vi "Tosca-Initialize Hardware.vi"(0 "Tosca":refnum<class "Parameters.lvclass">, 11 "error in (no error)":errorcluster) -> (4 "Tosca out":refnum<class "Parameters.lvclass">, 14 "SG Runtime":T1, 15 "error out":errorcluster)   [LabVIEW 2020]
uses:
  Typedefs/Tosca-SG Runtime Params.ctl
  Typedefs/Tosca-AO Runtime.ctl
  Typedefs/Tosca-DO Runtime.ctl
  Imaging VIs/Tosca-Imaging Mode.ctl
  Classes/Parameters/Parameters.lvclass
  epl-vi-lib/PXI DAQ VIs/AODO/Typedefs/AODO-Config.ctl
  epl-vi-lib/PXI DAQ VIs/AODO/Typedefs/AODO-Output Spec.ctl
  epl-vi-lib/PXI DAQ VIs/AODO/Typedefs/DO-Output Spec.ctl
  epl-vi-lib/PXI DAQ VIs/AODO/Typedefs/AODO-Action.ctl
  Imaging VIs/Tosca-2P Config.ctl
  Classes/Parameters/Parameters.lvclass/Parameters.ctl
  Classes/Parameters/Read Imaging.vi
  Classes/Parameters/Read DAQ.vi
  Tosca-Globals.vi
  epl-vi-lib/Utility VIs/File IO VIs/Configuration File Wrapper VIs/Config-Read Key (string).vi
  epl-vi-lib/Utility VIs/Array Manipulation VIs/Sort and Index (string).vi
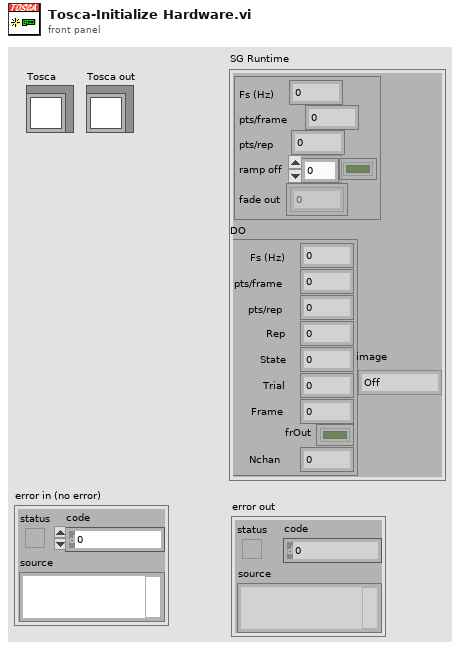
[diagram p1: front panel]
types:
  T1 = typedef "Tosca-SG Runtime Params.ctl" = cluster{"AO":T2, "DO":T3, "image":T4}
  T2 = typedef "Tosca-AO Runtime.ctl" = cluster{"Fs (Hz)":dbl, "pts/frame":i32, "pts/rep":i32, "ramp off":bool[], "fade out":dbl[][]}
  T3 = typedef "Tosca-DO Runtime.ctl" = cluster{"Fs (Hz)":dbl, "pts/frame":i32, "pts/rep":i32, "Rep":i32, "State":i32, "Trial":i32, "Frame":i32, "frOut":bool[], "Nchan":i32}
  T4 = typedef "Tosca-Imaging Mode.ctl" = enum16{"Off", "Widefield", "Two-photon"}
  T5 = typedef "AODO-Action.ctl" = enum16{"Configure", "Initialize", "Start", "Write", "Clean up", "Init & Start", "Config & Test", "Position", "Set AO Gains", "Zero", "Prime", "Status"}
  T6 = typedef "AODO-Config.ctl" = cluster{"AO":T7, "DO":T8, "hold outputs":bool, "ExtTrig":bool, "Trig Src":string, "regen":bool, "finite":bool}
  T7 = typedef "AODO-Output Spec.ctl" = cluster{"Channels":string[], "Fs (Hz)":dbl, "Npts":i32, "Gains":dbl[]}
  T8 = typedef "DO-Output Spec.ctl" = cluster{"Channels":string[], "Fs (Hz)":dbl, "Npts":i32, "Port":string}
  T9 = typedef "Tosca-2P Config.ctl" = cluster{"Frame tracker":string, "Terminal":string, "Trigger source":string}
  T10 = typedef "Tosca-Imaging.ctl" = cluster{"mode":T4, "FrameRateHz":dbl, "use AO":bool, "destination":string}
  T11 = typedef "Parameters.lvclass/DAQ.ctl" = cluster{"AO Fs (Hz)":dbl, "DO Fs (Hz)":dbl, "Poll Rate (Hz)":dbl, "Baseline (s)":dbl}
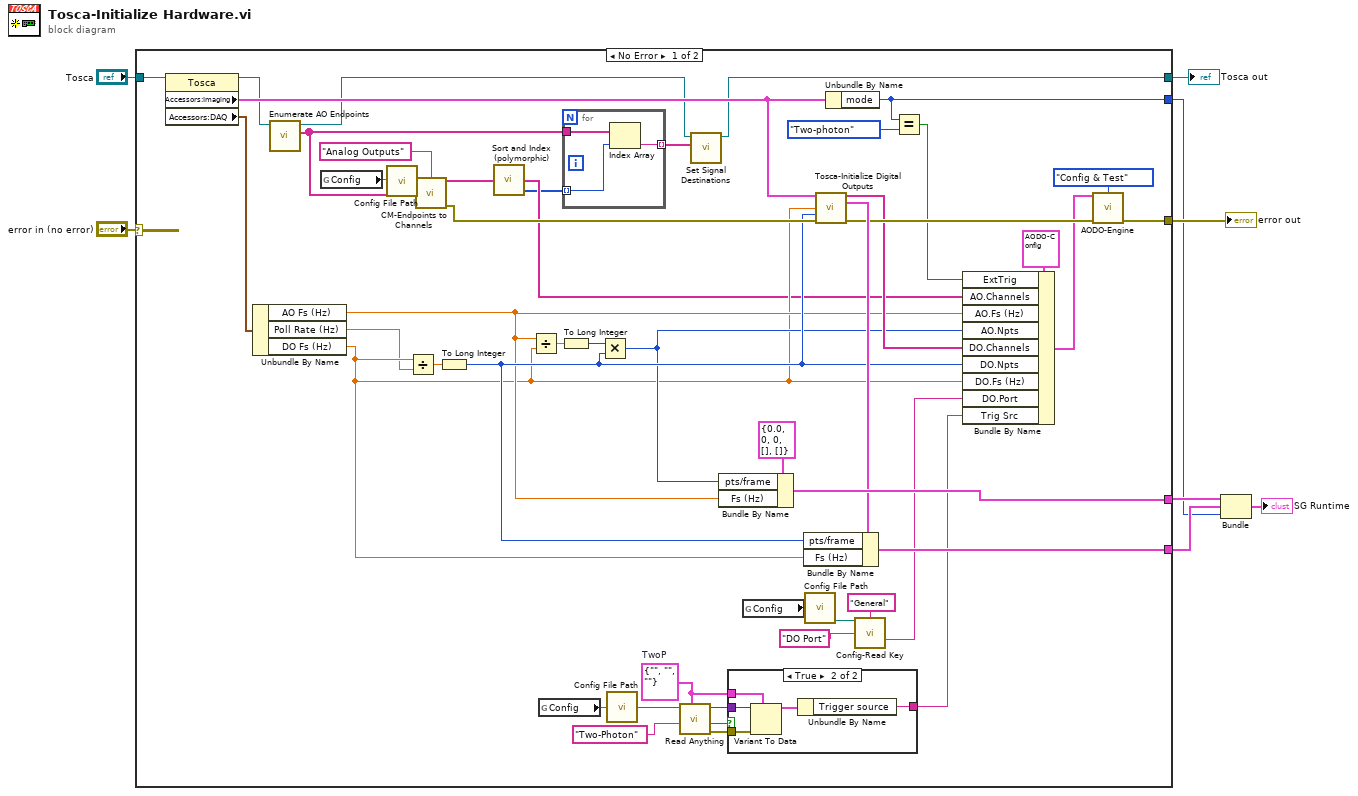
[diagram p0: block diagram]
diagram:
  n1 = case shown="No Error" "error in (no error)" {
    selector: "error in (no error)" -> [_ w67]
    tunnel: [w46 w67] -> w4
    tunnel: [w55 _] -> w7
    tunnel: [w54 _] -> w6
    tunnel: [w45 _] -> w3
    tunnel: "Tosca" -> [w23 w66]
    tunnel: [w11 w66] -> w1
    frame No Error {
      w30 = T9 {"Frame tracker"="", "Terminal"="", "Trigger source"=""}  # TwoP
      n2 = property class="Tosca"(reference=w23) -> (reference out=w18:refnum<class "Parameters.lvclass">, "Accessors:Imaging"=w22:T10, "Accessors:DAQ"=w21:T11)  [unwired: 1 in, 1 out]
      n3 = Unbundle By Name(w21) -> ("AO Fs (Hz)"=w20:dbl, "Poll Rate (Hz)"=w10:dbl, "DO Fs (Hz)"=w19:dbl)
      n4 = call "Enumerate AO Endpoints.vi"("Tosca in"=w18) -> ("Endpoints"=w14:string[], "Tosca out"=w12:refnum<class "Parameters.lvclass">)  [unwired: 8 in, 1 out]
      n5 = global read "Tosca-Globals.vi" "Config"() -> (w24:string)
      n6 = call "Config File Path.vi"("AppName"=w24) -> ("Default config file name"=w34:path)
      n7 = Divide(x=w19, y=w10) -> (x/y=w57:dbl)
      n8 = call "CM-Endpoints to Channels.vi"("Path"=w34, "IO Type"="Analog Outputs", "Requested Endpoints"=w14) -> ("IO Channels"=w17:string[], "error out"=w52:errorcluster)  [unwired: 11 in]
      n9 = To Long Integer(number=w57) -> (32bit integer=w39:i32)
      n10 = call-poly "Sort and Index (polymorphic).vi"("X"=w17) -> ("Index"=w15:i32[], "Sort(X)"=w16:string[])  [unwired: 3 in]
      n11 = Divide(x=w20, y=w19) -> (x/y=w38:dbl)
      n12 = global read "Tosca-Globals.vi" "Config"() -> (w26:string)
      n13 = To Long Integer(number=w38) -> (32bit integer=w36:i32)
      n14 = for {
        tunnel: w15 -> [w59] mode=indexing
        tunnel: w14 -> [w60]
        tunnel: [w58] -> w13 mode=indexing
        n15 = Index Array(array=w60, index=w59) -> (element=w58:string)
      }
      n16 = Multiply(x=w36, y=w39) -> (x*y=w37:i32)
      n17 = call "Config File Path.vi"("AppName"=w26) -> ("Default config file name"=w27:path)
      n18 = call "Read Anything.vi"("Type of Anything"=w30, "Section Name (Name of \"Type of Anything\")"="Two-Photon" ("Section Name (Name of \"Type of Anything\")"), "Path (dialog)"=w27) -> ("Error Out"=w31:errorcluster, "Found?"=w28:bool, "Anything"=w32:variant)  [unwired: 6 in]
      n19 = call "Set Signal Destinations.vi"("Endpoints"=w13, "Tosca in"=w12) -> ("Tosca out"=w11:refnum<class "Parameters.lvclass">)  [unwired: 8 in, 1 out]
      n20 = Bundle By Name(cluster=T2 {"Fs (Hz)"=0.0, "pts/frame"=0, "pts/rep"=0, "ramp off"=[], "fade out"=[]} ("Dummy Runtime"), "pts/frame"=w37, "Fs (Hz)"=w20) -> (w55:T2)
      n21 = case shown="True" w28 {
        tunnel: w32 -> [_ w65]
        tunnel: w31 -> [_ w64]
        tunnel: w30 -> [_ w63]
        tunnel: [_ w61] -> w29
        frame False {
        }
        frame True {
          n22 = Variant To Data(error in=w64, type=w63, Variant=w65) -> (data=w62:T9)  [unwired: 1 out]
          n23 = Unbundle By Name(w62) -> ("Trigger source"=w61:string)
        }
      }
      n24 = global read "Tosca-Globals.vi" "Config"() -> (w25:string)
      n25 = call "Config File Path.vi"("AppName"=w25) -> ("Default config file name"=w41:path)
      n26 = call "Tosca-Initialize Digital Outputs.vi"("Imaging"=w22, "Fs (Hz)"=w19, "Npts"=w39, "error in (no error)"=w52) -> ("Digital Outputs"=w47:string[], "DO"=w53:T3, "error out"=w50:errorcluster)  [unwired: 9 in]
      n27 = Bundle By Name(cluster=w53, "pts/frame"=w39, "Fs (Hz)"=w19) -> (w54:T3)
      n28 = Unbundle By Name(w22) -> ("mode"=w45:T4)
      n29 = call-poly "Config-Read Key.vi"("configuration file path"=w41, "section"="General", "key"="DO Port") -> ("value"=w40:string)  [unwired: 9 in, 3 out]
      n30 = Equal?(x=w45, y=Tosca-Imaging_Mode."Two-photon") -> (x = y?=w35:bool)
      n31 = Bundle By Name(cluster=T6 {"AO"={"Channels"=[], "Fs (Hz)"=0.0, "Npts"=0, "Gains"=[]}, "DO"={"Channels"=[], "Fs (Hz)"=0.0, "Npts"=0, "Port"=""}, "hold outputs"=FALSE, "ExtTrig"=FALSE, "Trig Src"="", "regen"=FALSE, "finite"=FALSE} ("Config"), "ExtTrig"=w35, "AO.Channels"=w16, "AO.Fs (Hz)"=w20, "AO.Npts"=w37, "DO.Channels"=w47, "DO.Npts"=w39, "DO.Fs (Hz)"=w19, "DO.Port"=w40, "Trig Src"=w29) -> (w49:T6)
      n32 = call "AODO-Engine.vi"("Config"=w49, "Action"=AODO-Action."Config & Test", "error in (no error)"=w50) -> ("error out"=w46:errorcluster)  [unwired: 7 in, 5 out]
    }
    frame Error {
    }
  }
  "error out" <- w4
  "Tosca out" <- w1
  n33 = Bundle("Dummy Runtime"=w7, "DO"=w6, "mode"=w3) -> (→"SG Runtime":cluster{"Dummy Runtime":T2, "DO":T3, "mode":T4})  [unwired: 1 in]
